vi "Charger_Append Reopen Status.vi"(5 "Status Refnum":T1, 6 "error in":errorcluster, 8 "NOT In Session":bool) -> (0 "error out":errorcluster {"code" format="%.0x"})   [LabVIEW 2020]
doc: "This function appends an \"IPG Shutdown successfully.\" message to the IPG Status cluster status field, if the \"idle\" flag is TRUE and the error status is clear."
uses:
  Charger_Status Refnum.ctl
  Drivers/Charger Test Set/Charger_Input Control.ctl
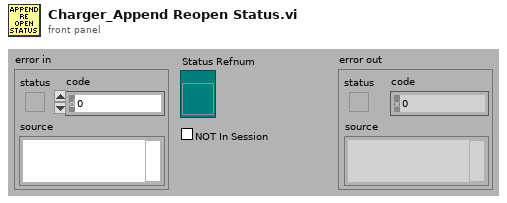
[diagram p1: front panel]
types:
  T1 = typedef "Charger_Status Refnum.ctl" = refnum<vi>
  T2 = typedef "Charger_Input Control.ctl" = cluster{"address":refnum<visa-resource-name>, "position":i32, "setpoint":dbl}
  T3 = cluster{"MICS ID":u32, "VBAT":dbl, "ChargingState":string, "VBAT Slide":dbl, "Status":string, "TemperatureLevel":dbl, "IPG_ReceivedLevel":dbl, "VBAT Target":dbl, "Charger Setpoint":dbl, "Index":i32, "Ready":bool, "Charger Inputs":T2, "MICS Inputs":cluster{"address":refnum<visa-resource-name>, "chan":u16, "ID":u32}}
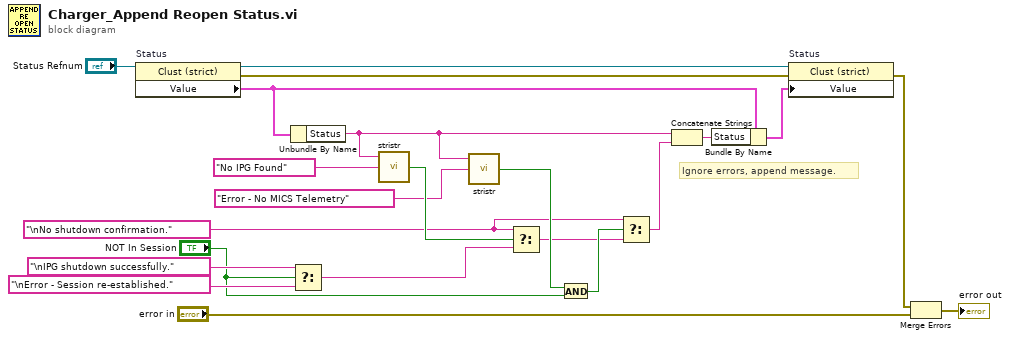
[diagram p0: block diagram]
diagram:
  w3 = "\nNo shutdown confirmation."
  # "Ignore errors, append message."
  n1 = property on="Status" class="Clust (strict)"(reference="Status Refnum") -> (reference out=w20:T1, error out=w21:errorcluster, "Value"=w19:T3)  [unwired: 1 in]
  n2 = Unbundle By Name(w19) -> ("Status"=w8:string)
  n3 = Select(t="\nIPG shutdown successfully." ("status message"), s="NOT In Session", f="\nError - Session re-established." ("status message")) -> (s? t:f=w11:string)
  n4 = call "stristr.vi"("Substring"="No IPG Found" ("regular expression"), "Input String"=w8) -> ("found"=w10:bool)  [unwired: 1 in, 2 out]
  n5 = call "stristr.vi"("Substring"="Error - No MICS Telemetry", "Input String"=w8) -> ("found"=w5:bool)  [unwired: 1 in, 2 out]
  n6 = Select(t=w3, s=w10, f=w11) -> (s? t:f=w2:string)
  n7 = And(x=w5, y="NOT In Session") -> (x .and. y?=w4:bool)
  n8 = Select(t=w3, s=w4, f=w2) -> (s? t:f=w1:string)
  n9 = Concatenate Strings(w8, w1) -> (w17:string)
  n10 = Bundle By Name(cluster=w19, "Status"=w17) -> (w18:T3)
  n11 = property on="Status" class="Clust (strict)"(reference=w20, error in=w21, "Value"=w18) -> (error out=w16:errorcluster)  [unwired: 1 out]
  n12 = Merge Errors(w16, "error in") -> (→"error out":errorcluster)
